vi "释放通道后申请通道.vi"(8 "error in":errorcluster, 10 "通道":string) -> (0 "error out":errorcluster)   [LabVIEW 2011]
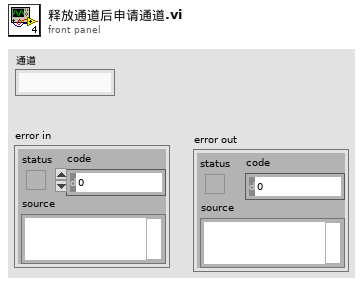
[diagram p1: front panel]
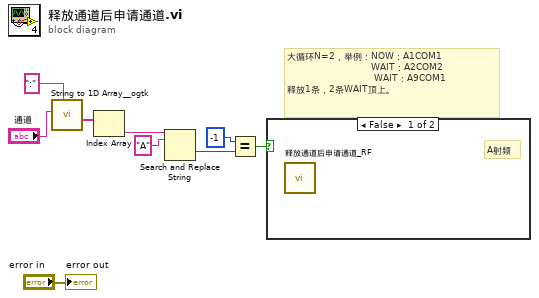
[diagram p0: block diagram]
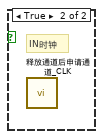
[diagram p2: hidden frame]
diagram:
  # "大循环N=2，举例：NOW：A1COM1\n                            WAIT：A2COM2\n                             WAIT：A9COM1\n释放1条，2条WAIT顶上。"
  n1 = call <userlib>:"String to 1D Array__ogtk.vi"("delimiter (Tab)"=":", "string"="通道") -> ("Array of Strings"=w8:string[])  [unwired: 9 in]
  n2 = Index Array(array=w8) -> (element=w3:string)  [unwired: 1 in]
  n3 = Search and Replace String(input string=w3, search string="A") -> (offset past replacement=w5:i32)  [unwired: 6 in, 3 out]
  n4 = Equal?(x=-1, y=w5) -> (x = y?=w2:bool)
  n5 = case shown="False" w2 {
    frame False {
      # "A射频"
      n6 = call "释放通道后申请通道_RF.vi"() -> ()  [unwired: 11 in, 1 out]
    }
    frame True {
      # "IN时钟"
      n7 = call "释放通道后申请通道_CLK.vi"() -> ()  [unwired: 11 in, 1 out]
    }
  }
  "error out" <- "error in"
